vi "Measurement.Free.UI.GetDependencies.vi"(8 "error in (no error)":errorcluster, 11 "Measurement.Free.UI in":refnum<class "Measurement.Free.UI.lvclass">) -> (0 "error out":errorcluster, 2 "Dependencies":T1, 3 "Measurement.Free.UI out":refnum<class "Measurement.Free.UI.lvclass">)   [LabVIEW 2017, in "Measurement.Free.UI.lvclass"]
uses:
  Measurement.Free.UI.lvclass
  Typedefs/Dependencies--Cluster.ctl
  Measurement.Free/Measurement.Free.lvclass
  Measurement.Free.UI.lvclass/Measurement.Free.UI.ctl
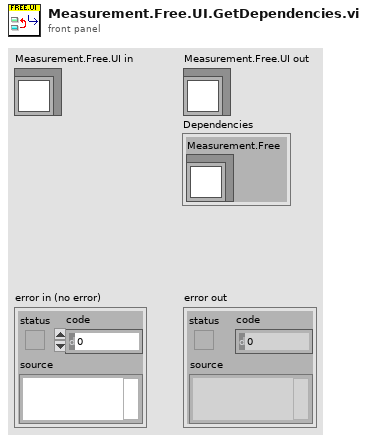
[diagram p1: front panel]
types:
  T1 = typedef "Measurement.Free.UI.lvclass/Dependencies--Cluster.ctl" = cluster{"Measurement.Free":refnum<class "Measurement.Free.lvclass">}
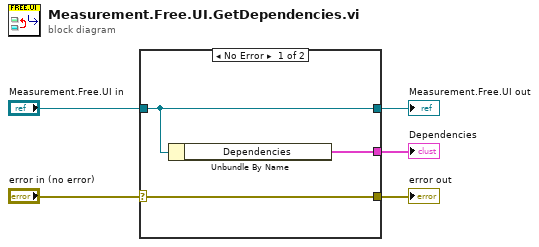
[diagram p0: block diagram]
diagram:
  n1 = case shown="No Error" "error in (no error)" {
    selector: "error in (no error)" -> [w8 w10]
    tunnel: [w8 w10] -> w4
    tunnel: [w7 w9] -> w2
    tunnel: "Measurement.Free.UI in" -> [w7 w9]
    tunnel: [w6 _] -> w1
    frame No Error {
      n2 = Unbundle By Name(w7) -> ("Dependencies"=w6:T1)
    }
    frame Error {
    }
  }
  "error out" <- w4
  "Measurement.Free.UI out" <- w2
  "Dependencies" <- w1
